vi "RxBfrPkt - Init Packet Page.vi"(6 "Rx Buffered Data Packet Refs":T1, 8 "error in (no error)":errorcluster, 11 "Node Ptr In":T2 format="%.0x") -> (0 "error out":errorcluster, 3 "Node Ptr Out":T2 format="%.0x")   [LabVIEW 2019, in "UDP-Custom-Device System Explorer.lvlib"]
uses:
  UDP-Custom-Device System Explorer.lvlib
  <vilib>/NI VeriStand/Custom Device API/Custom Device Item Ref.ctl
  Types/Page References/Refs - Rx Buffered Data Packet Page.ctl
  Property Accessors/Buffered Data Packet.lvlib
  Property Accessors/Shared Packet Accessors.lvlib
  <vilib>/NI VeriStand/Custom Device API/Custom Device API.lvlib
  Property Accessors/Rx Packet Accessors.lvlib
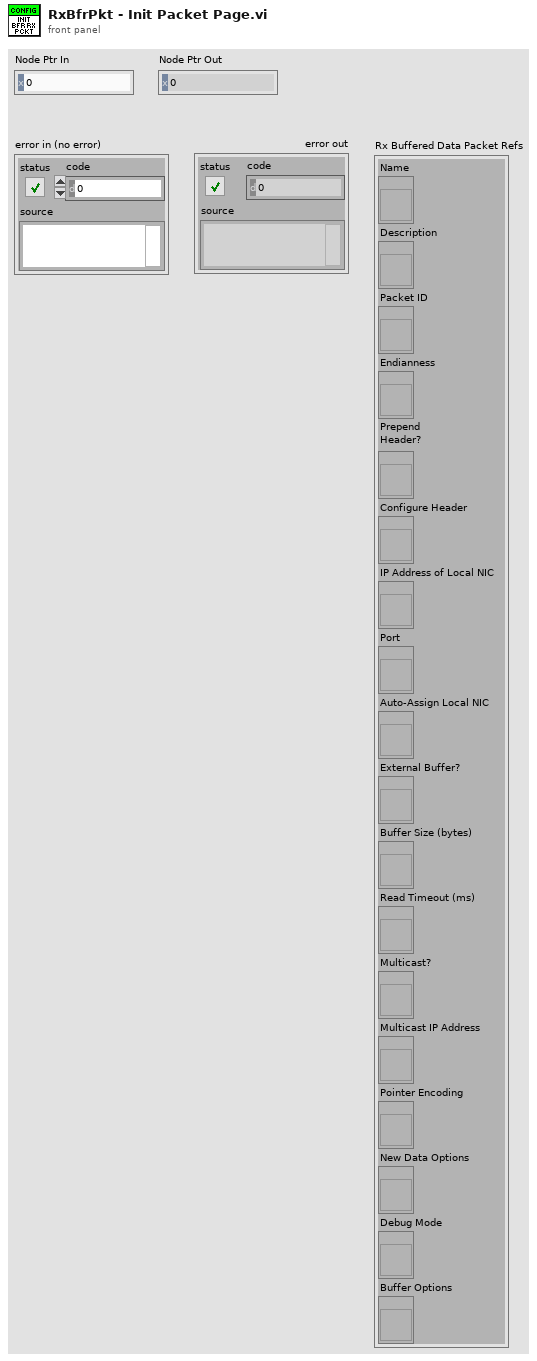
[diagram p1: front panel]
types:
  T1 = typedef "UDP-Custom-Device System Explorer.lvlib/Refs - Rx Buffered Data Packet Page.ctl" = cluster{"Name":refnum<vi>, "Description":refnum<vi>, "Packet ID":refnum<vi>, "Endianness":refnum<vi>, "Prepend\nHeader?":refnum<vi>, "Configure Header":refnum<vi>, "IP Address of Local NIC":refnum<vi>, "Port":refnum<vi>, "Auto-Assign Local NIC":refnum<vi>, "External Buffer?":refnum<vi>, "Buffer Size (bytes)":refnum<vi>, "Read Timeout (ms)":refnum<vi>, "Multicast?":refnum<vi>, "Multicast IP Address":refnum<vi>, "Pointer Encoding":refnum<vi>, "New Data Options":refnum<vi>, "Debug Mode":refnum<vi>, "Buffer Options":refnum<vi>}
  T2 = typedef "Custom Device API.lvlib/Custom Device Item Ref.ctl" = u64
  T3 = enum8{"Enabled", "Disabled", "Disabled and Grayed Out"}
  T4 = typedef "UDP-Custom-Device Shared.lvlib/Shared - Receive Buffer Options.ctl" = enum16{"Static Buffer", "Circular Buffer", "Circular Buffer + Size", "Internal Cache", "Internal Cache + Size", "Ping Pong", "Ping Pong + Size"}
  T5 = typedef "UDP-Custom-Device Shared.lvlib/Shared - New Data Options.ctl" = enum16{"Timeout Reset", "Counter"}
  T6 = typedef "UDP-Custom-Device Shared.lvlib/Shared - Pointer Encoding.ctl" = enum16{"Direct Encoding", "Conversion Encoding"}
  T7 = typedef "Custom Device API.lvlib/Custom Device Item Info.ctl" = cluster{"Name":string, "Is Channel":bool, "GUID":string, "Is Waveform":bool}
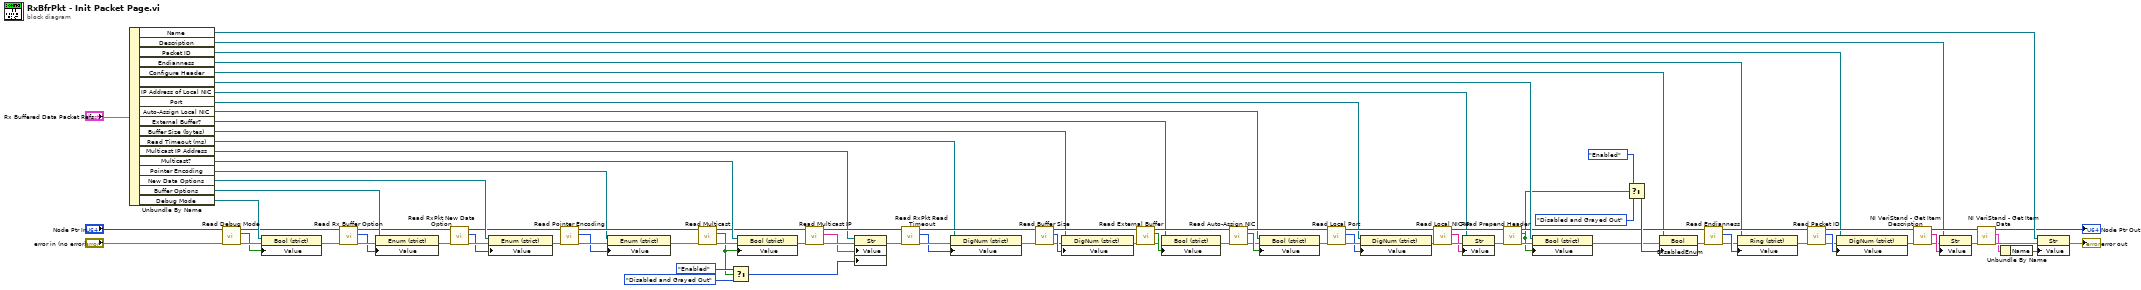
[diagram p0: block diagram]
diagram:
  n1 = Unbundle By Name("Rx Buffered Data Packet Refs") -> ("Name"=w43:refnum<vi>, "Description"=w44:refnum<vi>, "Packet ID"=w45:refnum<vi>, "Endianness"=w46:refnum<vi>, "Configure Header"=w47:refnum<vi>, "Prepend\nHeader?"=w70:refnum<vi>, "IP Address of Local NIC"=w71:refnum<vi>, "Port"=w72:refnum<vi>, "Auto-Assign Local NIC"=w73:refnum<vi>, "External Buffer?"=w74:refnum<vi>, "Buffer Size (bytes)"=w75:refnum<vi>, "Read Timeout (ms)"=w39:refnum<vi>, "Multicast IP Address"=w30:refnum<vi>, "Multicast?"=w35:refnum<vi>, "Pointer Encoding"=w21:refnum<vi>, "New Data Options"=w17:refnum<vi>, "Buffer Options"=w12:refnum<vi>, "Debug Mode"=w7:refnum<vi>)
  n2 = call "Read Debug Mode.vi"("error in (no error)"="error in (no error)", "Node Ptr"="Node Ptr In") -> ("error out"=w2:errorcluster, "Debug Mode"=w1:bool, "Node Ptr out"=w4:T2)  [unwired: 7 in]
  n3 = property class="Bool (strict)"(reference=w7, error in=w2, "Value"=w1) -> (error out=w6:errorcluster)  [unwired: 1 out]
  n4 = call "Read Rx Buffer Option.vi"("error in (no error)"=w6, "Node Ptr"=w4) -> ("error out"=w10:errorcluster, "Buffer Option"=w8:T4, "Node Ptr out"=w9:T2)  [unwired: 7 in]
  n5 = property class="Enum (strict)"(reference=w12, error in=w10, "Value"=w8) -> (error out=w11:errorcluster)  [unwired: 1 out]
  n6 = call "Read RxPkt New Data Option.vi"("error in (no error)"=w11, "Node Ptr"=w9) -> ("error out"=w14:errorcluster, "New Data Option"=w13:T5, "Node Ptr out"=w15:T2)  [unwired: 7 in]
  n7 = property class="Enum (strict)"(reference=w17, error in=w14, "Value"=w13) -> (error out=w16:errorcluster)  [unwired: 1 out]
  n8 = call "Read Pointer Encoding.vi"("error in (no error)"=w16, "Node Ptr"=w15) -> ("error out"=w20:errorcluster, "Pointer Encoding"=w18:T6, "Node Ptr out"=w22:T2)  [unwired: 7 in]
  n9 = property class="Enum (strict)"(reference=w21, error in=w20, "Value"=w18) -> (error out=w19:errorcluster)  [unwired: 1 out]
  n10 = call "Read Multicast.vi"("error in (no error)"=w19, "Node Ptr"=w22) -> ("error out"=w34:errorcluster, "Multicast"=w24:bool, "Node Ptr out"=w32:T2)  [unwired: 7 in]
  n11 = Select(t=T3."Enabled" ("Disabled"), s=w24, f=T3."Disabled and Grayed Out" ("Disabled")) -> (s? t:f=w23:T3)
  n12 = property class="Bool (strict)"(reference=w35, error in=w34, "Value"=w24) -> (error out=w33:errorcluster)  [unwired: 1 out]
  n13 = call "Read Multicast IP.vi"("error in (no error)"=w33, "Node Ptr"=w32) -> ("error out"=w29:errorcluster, "Multicast IP Address"=w27:string, "Node Ptr out"=w31:T2)  [unwired: 7 in]
  n14 = property class="Str"(reference=w30, error in=w29, "Value"=w27, "DisabledEnum"=w23) -> (error out=w28:errorcluster)  [unwired: 1 out]
  n15 = call "Read RxPkt Read Timeout.vi"("error in (no error)"=w28, "Node Ptr"=w31) -> ("error out"=w38:errorcluster, "Read Timeout"=w36:i32, "Node Ptr out"=w40:T2)  [unwired: 7 in]
  n16 = property class="DigNum (strict)"(reference=w39, error in=w38, "Value"=w36) -> (error out=w37:errorcluster)  [unwired: 1 out]
  n17 = call "Read Buffer Size.vi"("error in (no error)"=w37, "Node Ptr"=w40) -> ("error out"=w95:errorcluster, "Buffer Size"=w96:u32, "Node Ptr out"=w90:T2)  [unwired: 7 in]
  n18 = property class="DigNum (strict)"(reference=w75, error in=w95, "Value"=w96) -> (error out=w92:errorcluster)  [unwired: 1 out]
  n19 = call "Read External Buffer.vi"("error in (no error)"=w92, "Node Ptr"=w90) -> ("error out"=w93:errorcluster, "External Buffer"=w94:bool, "Node Ptr out"=w91:T2)  [unwired: 7 in]
  n20 = property class="Bool (strict)"(reference=w74, error in=w93, "Value"=w94) -> (error out=w89:errorcluster)  [unwired: 1 out]
  n21 = call "Read Auto-Assign NIC.vi"("error in (no error)"=w89, "Node Ptr"=w91) -> ("error out"=w87:errorcluster, "Auto-Assign NIC"=w88:bool, "Node Ptr out"=w79:T2)  [unwired: 7 in]
  n22 = property class="Bool (strict)"(reference=w73, error in=w87, "Value"=w88) -> (error out=w78:errorcluster)  [unwired: 1 out]
  n23 = call "Read Local Port.vi"("error in (no error)"=w78, "Node Ptr"=w79) -> ("error out"=w85:errorcluster, "Port"=w84:u16, "Node Ptr out"=w86:T2)  [unwired: 7 in]
  n24 = property class="DigNum (strict)"(reference=w72, error in=w85, "Value"=w84) -> (error out=w83:errorcluster)  [unwired: 1 out]
  n25 = call "Read Local NIC IP.vi"("error in (no error)"=w83, "Node Ptr"=w86) -> ("error out"=w82:errorcluster, "IP Address of Local NIC"=w81:string, "Node Ptr out"=w76:T2)  [unwired: 7 in]
  n26 = property class="Str"(reference=w71, error in=w82, "Value"=w81) -> (error out=w77:errorcluster)  [unwired: 1 out]
  n27 = call "Read Prepend Header.vi"("error in (no error)"=w77, "Node Ptr"=w76) -> ("error out"=w80:errorcluster, "Prepend Header"=w48:bool, "Node Ptr out"=w50:T2)  [unwired: 7 in]
  n28 = property class="Bool (strict)"(reference=w70, error in=w80, "Value"=w48) -> (error out=w49:errorcluster)  [unwired: 1 out]
  n29 = Select(t=T3."Enabled" ("Disabled"), s=w48, f=T3."Disabled and Grayed Out" ("Disabled")) -> (s? t:f=w69:T3)
  n30 = property class="Bool"(reference=w47, error in=w49, "DisabledEnum"=w69) -> (error out=w68:errorcluster)  [unwired: 1 out]
  n31 = call "Read Endianness.vi"("error in (no error)"=w68, "Node Ptr"=w50) -> ("error out"=w63:errorcluster, "Endianness"=w64:u16, "Node Ptr out"=w65:T2)  [unwired: 7 in]
  n32 = property class="Ring (strict)"(reference=w46, error in=w63, "Value"=w64) -> (error out=w62:errorcluster)  [unwired: 1 out]
  n33 = call "Read Packet ID.vi"("error in (no error)"=w62, "Node Ptr"=w65) -> ("error out"=w60:errorcluster, "Packet ID"=w61:i32, "Node Ptr out"=w59:T2)  [unwired: 7 in]
  n34 = property class="DigNum (strict)"(reference=w45, error in=w60, "Value"=w61) -> (error out=w58:errorcluster)  [unwired: 1 out]
  n35 = call <vilib>:"NI VeriStand - Get Item Description.vi"("error in (no error)"=w58, "Item Ref in"=w59) -> ("error out"=w53:errorcluster, "Description"=w54:string, "Item Ref out"=w56:T2)  [unwired: 7 out]
  n36 = property class="Str"(reference=w44, error in=w53, "Value"=w54) -> (error out=w55:errorcluster)  [unwired: 1 out]
  n37 = call <vilib>:"NI VeriStand - Get Item Data.vi"("error in (no error)"=w55, "Item Ref in"=w56) -> ("error out"=w52:errorcluster, "Item Info"=w51:T7, "Item Ref out"=→"Node Ptr Out":T2)  [unwired: 6 in, 1 out]
  n38 = Unbundle By Name(w51) -> ("Name"=w57:string)
  n39 = property class="Str"(reference=w43, error in=w52, "Value"=w57) -> (error out=→"error out":errorcluster)  [unwired: 1 out]
